vi "Revert LVClassLibrary Tools.vi"(11 "Files Installed":path[](array[path])) -> ()   [LabVIEW 2020]
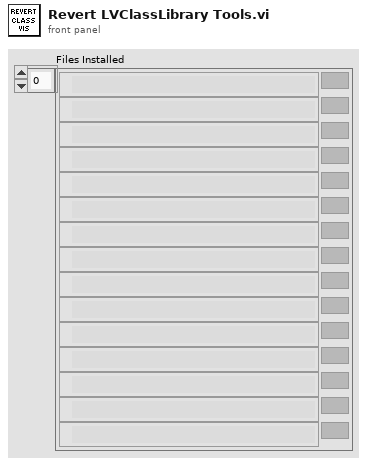
[diagram p1: front panel]
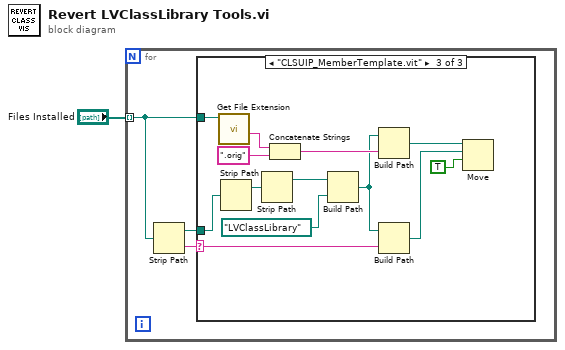
[diagram p0: block diagram]
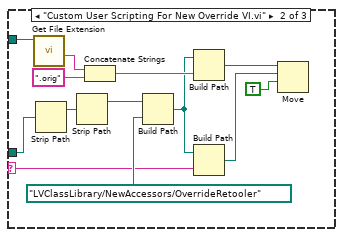
[diagram p3: hidden frame]
diagram:
  n1 = for {
    tunnel: "Files Installed" -> [w3] mode=indexing
    n2 = Strip Path(path=w3) -> (stripped path=w2:path, name=w4:string)
    n3 = case shown="\"CLSUIP_MemberTemplate.vit\"" w4 {
      selector: w4 -> [_ w5 w23]
      tunnel: w3 -> [_ w7 w28]
      tunnel: w2 -> [_ w6 w30]
      frame Default {
      }
      frame "Custom User Scripting For New Override VI.vi" {
        n4 = call <vilib>:"Get File Extension.vi"("file"=w7) -> ("filename without extension"=w16:string)  [unwired: 6 in, 4 out]
        n5 = Strip Path(path=w6) -> (stripped path=w17:path)  [unwired: 1 out]
        n6 = Strip Path(path=w17) -> (stripped path=w14:path)  [unwired: 1 out]
        n7 = Concatenate Strings(w16, ".orig" ("string")) -> (w12:string)
        n8 = Build Path(base path=w14, name or relative path=path "LVClassLibrary/NewAccessors/OverrideRetooler") -> (appended path=w11:path)
        n9 = Build Path(base path=w11, name or relative path=w12) -> (appended path=w10:path)
        n10 = Build Path(base path=w11, name or relative path=w5) -> (appended path=w9:path)
        n11 = Move(source path=w10, 9:TRUE ("overwrite (F)"), 10:w9) -> ()  [unwired: 2 in, 3 out]
      }
      frame "CLSUIP_MemberTemplate.vit" {
        n12 = call <vilib>:"Get File Extension.vi"("file"=w28) -> ("filename without extension"=w27:string)  [unwired: 6 in, 4 out]
        n13 = Strip Path(path=w30) -> (stripped path=w29:path)  [unwired: 1 out]
        n14 = Strip Path(path=w29) -> (stripped path=w25:path)  [unwired: 1 out]
        n15 = Concatenate Strings(w27, ".orig" ("string")) -> (w22:string)
        n16 = Build Path(base path=w25, name or relative path=path "LVClassLibrary") -> (appended path=w21:path)
        n17 = Build Path(base path=w21, name or relative path=w22) -> (appended path=w20:path)
        n18 = Build Path(base path=w21, name or relative path=w23) -> (appended path=w19:path)
        n19 = Move(source path=w20, 9:TRUE ("overwrite (F)"), 10:w19) -> ()  [unwired: 2 in, 3 out]
      }
    }
  }
